vi "Close Log File.vi"(8 "error in (no error)":errorcluster, 11 "Log Producer in":refnum<class "Log Producer.lvclass">) -> (0 "error out":errorcluster, 3 "Log Producer out":refnum<class "Log Producer.lvclass">)   [LabVIEW 2020, in "AIM MIL-STD-1553 Engine.lvlib" / "Implementation.lvlib" / "Word Logging.lvlib" / "Log Producer.lvclass"]
uses:
  Log Producer.lvclass
  Log Producer.lvclass/Log Producer.ctl
  Logger Interface/Logger Interface.lvclass
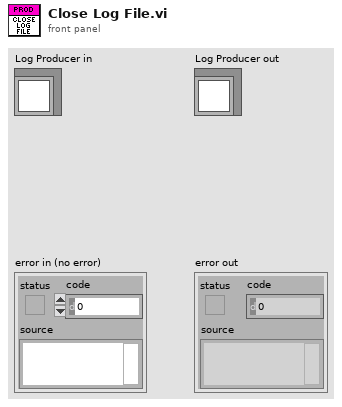
[diagram p1: front panel]
types:
  T1 = typedef "AIM MIL-STD-1553 Engine.lvlib/Implementation.lvlib/Word Logging.lvlib/Logger Data Reference.ctl" = refnum<data-value>
  T2 = cluster{"Logger Interface":refnum<class "Logger Interface.lvclass">}
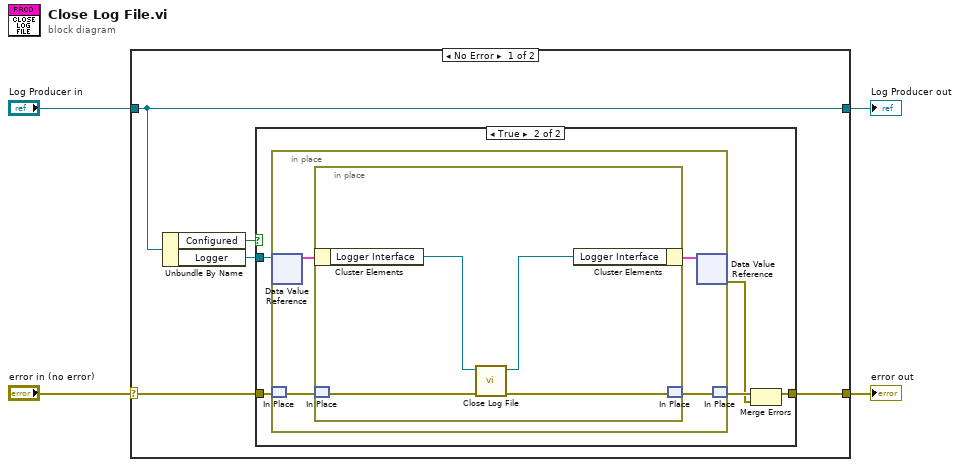
[diagram p0: block diagram]
diagram:
  n1 = case shown="No Error" "error in (no error)" {
    selector: "error in (no error)" -> [w9 w25]
    tunnel: [w6 w25] -> w3
    tunnel: [w8 w24] -> w1
    tunnel: "Log Producer in" -> [w8 w24]
    frame No Error {
      n2 = Unbundle By Name(w8) -> ("Configured"=w5:bool, "Logger"=w7:T1)
      n3 = case shown="True" w5 {
        tunnel: w9 -> [w10 w15]
        tunnel: w7 -> [_ w14]
        tunnel: [w10 w12] -> w6
        frame False {
        }
        frame True {
          n4 = in-place {
            n5 = in-place-dvr #1(w14) -> (w17:T2)  [unwired: 1 out]
            n6 = in-place-match #2(w15) -> (w19:errorcluster)
            n7 = in-place {
              n8 = in-place-cluster #3(w17) -> ("Logger Interface"=w21:refnum<class "Logger Interface.lvclass">)
              n9 = in-place-match #4(w19) -> (w23:errorcluster)
              n10 = call-dynamic "Close Log File.vi"("error in (no error)"=w23, "Logger Interface in"=w21) -> ("error out"=w22:errorcluster, "Logger Interface out"=w20:refnum<class "Logger Interface.lvclass">)  [unwired: 8 in]
              n11 = in-place-cluster #3("Logger Interface"=w20) -> (w16:T2)
              n12 = in-place-match #4(w22) -> (w18:errorcluster)
            }
            n13 = in-place-dvr #1(w16) -> (w11:errorcluster)  [unwired: 1 out]
            n14 = in-place-match #2(w18) -> (w13:errorcluster)
          }
          n15 = Merge Errors(w13, w11) -> (w12:errorcluster)
        }
      }
    }
    frame Error {
    }
  }
  "error out" <- w3
  "Log Producer out" <- w1
